vi "Waveform Peak Detection for 1 Chan.vi"(4 "end of data (T)":bool=TRUE, 6 "initialize (T)":bool=TRUE, 7 "peaks/valleys":u16(ring) items=["Peaks", "Valleys"], 8 "error in":errorcluster, 9 "width":i32=3 min=3, 10 "threshold":dbl format="%.2p", 11 "Signal In":waveform(dbl)) -> (0 "error out":errorcluster, 1 "2nd Derivatives":dbl[](array[numeric]) format="%.2p", 2 "Amplitudes":dbl[](array[numeric]) format="%.2p", 3 "Locations":dbl[](array[numeric]) format="%.2p", 5 "# found":i32)   [LabVIEW 2020, in "NI_MAPro.lvlib"]
doc: "Finds the locations, amplitudes, and second derivatives of peaks and valleys in <B>Signal In</B>. Wire data to the <B>Signal In</B> input to determine the polymorphic instance to use or manually select the instance."
uses:
  NI_MAPro.lvlib
  NI_MABase.lvlib
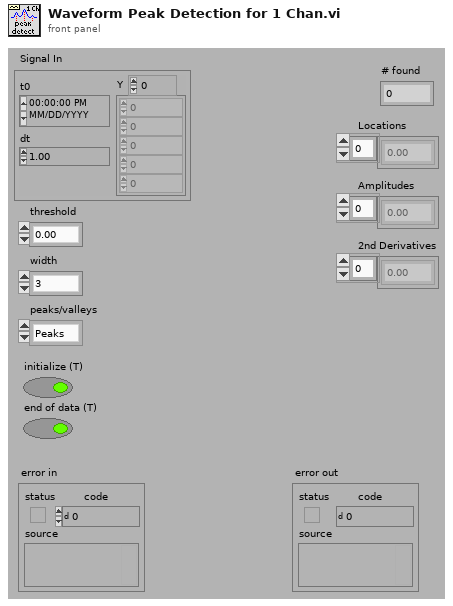
[diagram p1: front panel]
types:
  T1 = cluster{"PEAKINT":cluster{"Span":i32, "Index":i32, "NHistoryPts":i32, "Len":i32, "PrevSign":i32, "unused":i32, "RinvQt (pointer)":u32, "FitBuffer (pointer)":u32, "History (pointer)":u32, "PrevCoeff (pointer)":u32, "Data (pointer)":u32, "slack for RinvQt":u32, "slack for FitBuffer":u32, "slack for History":u32, "slack for PrevCoeff":u32, "slack for Data":u32}, "SavedData":dbl[]}
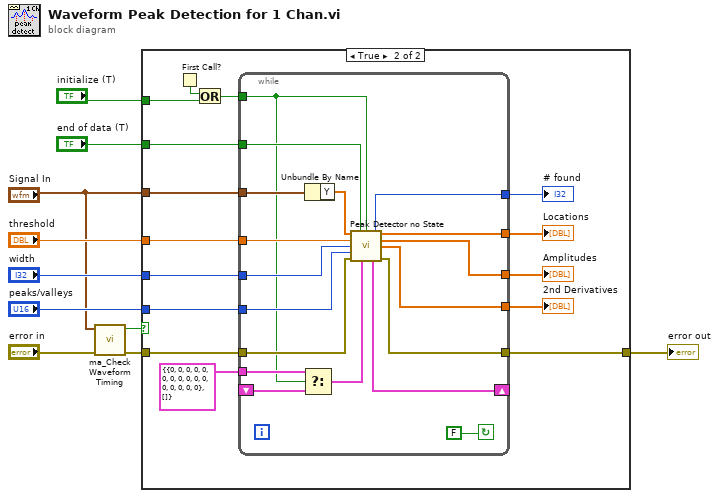
[diagram p0: block diagram]
diagram:
  n1 = call "ma_Check Waveform Timing.vi"("error in (no error)"="error in", "signal in"="Signal In") -> ("error out"=w3:errorcluster, "timing ok"=w2:bool)  [unwired: 1 in, 7 out]
  n2 = case shown="True" w2 {
    tunnel: w3 -> [w11 w26]
    tunnel: "threshold" -> [_ w25]
    tunnel: "peaks/valleys" -> [_ w24]
    tunnel: "end of data (T)" -> [_ w23]
    tunnel: "width" -> [_ w18]
    tunnel: "initialize (T)" -> [_ w17]
    tunnel: "Signal In" -> [_ w14]
    tunnel: [w11 w13] -> w1
    frame False {
    }
    frame True {
      n3 = First Call?() -> (First Call?: T/F=w16:bool)
      n4 = Or(x=w16, y=w17) -> (x .or. y?=w15:bool)
      n5 = while {
        tunnel: w26 -> [w44]
        tunnel: w25 -> [w43]
        tunnel: w24 -> [w42]
        tunnel: w15 -> [w28]
        tunnel: w23 -> [w41]
        tunnel: [w40] -> w22
        tunnel: [w39] -> w21
        tunnel: [w38] -> w20
        tunnel: [w37] -> w19
        tunnel: w18 -> [w36]
        tunnel: [w35] -> w13
        tunnel: w14 -> [w34]
        shift-right: [w31] -> _
        shift-left: _ -> [w29]
        tunnel: T1 {"PEAKINT"={"Span"=0, "Index"=0, "NHistoryPts"=0, "Len"=0, "PrevSign"=0, "unused"=0, "RinvQt (pointer)"=0, "FitBuffer (pointer)"=0, "History (pointer)"=0, "PrevCoeff (pointer)"=0, "Data (pointer)"=0, "slack for RinvQt"=0, "slack for FitBuffer"=0, "slack for History"=0, "slack for PrevCoeff"=0, "slack for Data"=0}, "SavedData"=[]} ("state info") -> [w30]
        stop <- FALSE continue-if-true
        n6 = Select(t=w30, s=w28, f=w29) -> (s? t:f=w27:T1)
        n7 = Unbundle By Name(w34) -> ("Y"=w33:dbl[])
        n8 = call "Peak Detector no State.vi"("X"=w33, "end of data (T)"=w41, "initialize (T)"=w28, "threshold"=w43, "width"=w36, "peaks/valleys"=w42, "error in"=w44, "state info"=w27) -> ("# found"=w37:i32, "Locations"=w40:dbl[], "Amplitudes"=w39:dbl[], "2nd Derivatives"=w38:dbl[], "state info"=w31:T1, "error out"=w35:errorcluster)  [unwired: 2 out]
      }
      "Locations" <- w22
      "Amplitudes" <- w21
      "2nd Derivatives" <- w20
      "# found" <- w19
    }
  }
  "error out" <- w1
